vi "Start Date and Time.vi"(1 "Search Detail":string, 2 "String IN":string) -> (0 "Header Detail":string)   [LabVIEW 2021]
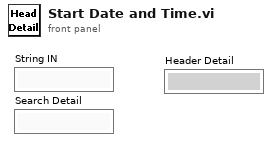
[diagram p1: front panel]
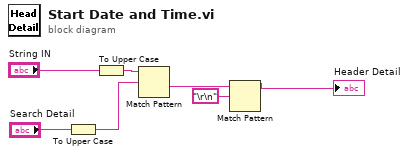
[diagram p0: block diagram]
diagram:
  n1 = To Upper Case(1:"Search Detail") -> (0:w2:string)
  n2 = To Upper Case(1:"String IN") -> (0:w3:string)
  n3 = Match Pattern(string=w3, regular expression=w2) -> (after substring=w4:string)  [unwired: 1 in, 3 out]
  n4 = Match Pattern(string=w4, regular expression="\r\n") -> (before substring=→"Header Detail":string)  [unwired: 1 in, 3 out]
